vi "numCmd_Recv_TwoDbl.vi"(7 "Command Name":string, 10 "Initial Value 2":dbl, 11 "Initial Value 1":dbl) -> (0 "error out":errorcluster, 1 "Any Changed":bool, 2 "Value 2":dbl, 3 "Value 1":dbl)   [LabVIEW 2019, in "Trajectory_Library.lvlib"]
uses:
  Trajectory_Library.lvlib
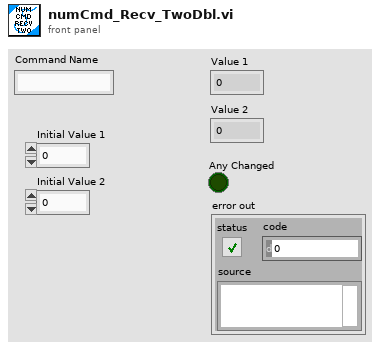
[diagram p1: front panel]
types:
  T1 = cluster{"Initial Value 1":dbl, "Initial Value 2":dbl}
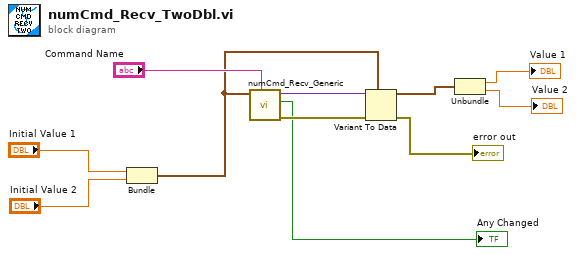
[diagram p0: block diagram]
diagram:
  n1 = Bundle("Initial Value 1"="Initial Value 1", "Initial Value 2"="Initial Value 2") -> (w3:T1)  [unwired: 1 in]
  n2 = call "numCmd_Recv_Generic.vi"("Command Name"="Command Name", "Initial Value"=w3) -> ("error out"=w11:errorcluster, "Changed"=→"Any Changed":bool, "Newest Value"=w2:variant)  [unwired: 7 in]
  n3 = Variant To Data(error in=w11, type=w3, Variant=w2) -> (data=w7:T1, error out=→"error out":errorcluster)
  n4 = Unbundle(w7) -> ("Initial Value 1"=→"Value 1":dbl, "Initial Value 2"=→"Value 2":dbl)
